vi "DWF FGEN Query Standard Waveform.vi"(0 "Instrument Handle In":u32, 11 "Error In":errorcluster caption="Error In (no error)") -> (2 "Duty Cycle":dbl, 3 "Frequency":dbl, 4 "Instrument Handle Out":u32, 6 "Waveform Function":i32(ring) items=["Sine", "Square", "Triangle/Ramp", "DC"], 8 "Amplitude":dbl, 10 "DC Offset":dbl, 15 "Error Out":errorcluster)   [LabVIEW 2015, in "DigilentWF.lvlib"]
doc: "Returns the settings for a standard waveform generation."
uses:
  <vilib>/DigilentWF/DigilentWF.lvlib
  dwf.dll
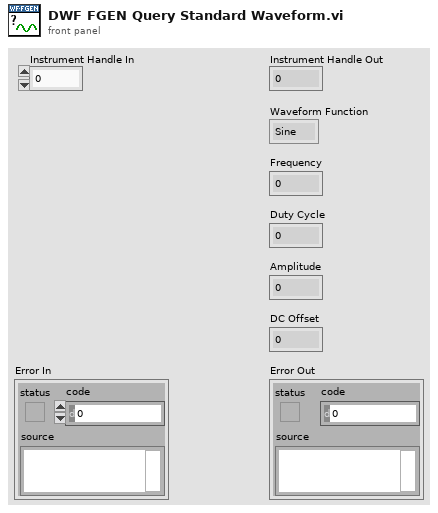
[diagram p1: front panel]
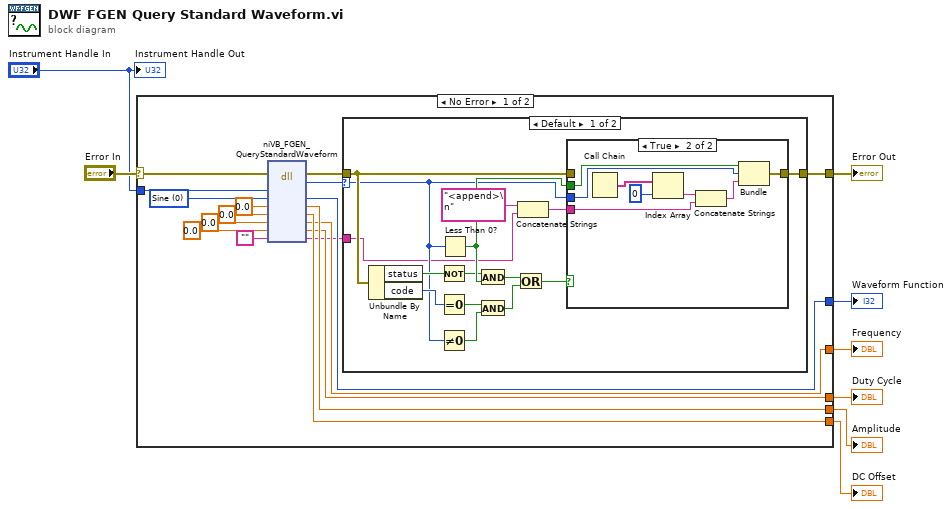
[diagram p0: block diagram]
diagram:
  n1 = case "outter_case" shown="No Error" "Error In" {
    selector: "Error In" -> [w24 w51]
    tunnel: [w25 w51] -> w7
    tunnel: "Instrument Handle In" -> [w23 _]
    tunnel: [w18 _] -> w5
    tunnel: [w15 _] -> w4
    tunnel: [w14 _] -> w3
    tunnel: [w17 _] -> w2
    tunnel: [w16 _] -> w1
    frame No Error {
      w22 = 0 items=["Sine", "Square", "Triangle/Ramp", "DC"] ("Waveform Function")
      n2 = dll-call lib="dwf.*" fn="niVB_FGEN_QueryStandardWaveform"(error in=w24, "instrumentHandle"=w23, "waveformFunction"=w22, "amplitude"=0.0 ("Frequency"), "dcOffset"=0.0 ("Duty Cycle"), "frequency"=0.0 ("Amplitude"), "dutyCycle"=0.0 ("DC Offset"), "szError"="") -> (error out=w20:errorcluster, "return type"=w19:i32, "waveformFunction"=w18:u32, "amplitude"=w17:dbl, "dcOffset"=w16:dbl, "frequency"=w15:dbl, "dutyCycle"=w14:dbl, "szError"=w9:string)  [unwired: 3 in, 1 out]
      n3 = case "inner_case" shown="Default" w19 {
        selector: w19 -> [w30 _]
        tunnel: w20 -> [w31 w50]
        tunnel: [w27 w50] -> w25
        tunnel: w9 -> [w26 _]
        frame Default {
          n4 = Unbundle By Name(w31) -> ("status"=w35:bool, "code"=w39:i32)
          n5 = Not(x=w35) -> (.not. x?=w38:bool)
          n6 = Equal To 0?(x=w39) -> (x = 0?=w34:bool)
          n7 = Not Equal To 0?(x=w30) -> (x != 0?=w37:bool)
          n8 = Less Than 0?(x=w30) -> (x < 0?=w40:bool)
          n9 = And(x=w38, y=w40) -> (x .and. y?=w36:bool)
          n10 = And(x=w34, y=w37) -> (x .and. y?=w33:bool)
          n11 = Or(x=w36, y=w33) -> (x .or. y?=w32:bool)
          n12 = Concatenate Strings("<append>\n" ("string"), w26) -> (w29:string)
          n13 = case shown="True" w32 {
            tunnel: [w41 w48] -> w27
            tunnel: w30 -> [_ w47]
            tunnel: w40 -> [_ w46]
            tunnel: w31 -> [w41 _]
            tunnel: w29 -> [_ w42]
            frame False {
            }
            frame True {
              n14 = Call Chain() -> (call chain=w45:string[])
              n15 = Index Array(array=w45, index=0) -> (element=w44:string)
              n16 = Concatenate Strings(w44, w42) -> (w49:string)
              n17 = Bundle(w46, "return type"=w47, w49) -> (w48:cluster{bool, "return type":i32, string})  [unwired: 1 out]
            }
          }
        }
        frame 0 {
        }
      }
    }
    frame Error {
    }
  }
  "Error Out" <- w7
  "Waveform Function" <- w5
  "Frequency" <- w4
  "Duty Cycle" <- w3
  "Amplitude" <- w2
  "DC Offset" <- w1
  "Instrument Handle Out" <- "Instrument Handle In"
